vi "IPC Flasher Main.vi"() -> ()   [LabVIEW 2021]
uses:
  Controls/Console Manager Functions.ctl
  SubVIs/Global Variable.vi
panel:
  out "Console":string
  in  "Barcode":string="Barcode"
  in  "Run":bool
  in  "Stop":bool
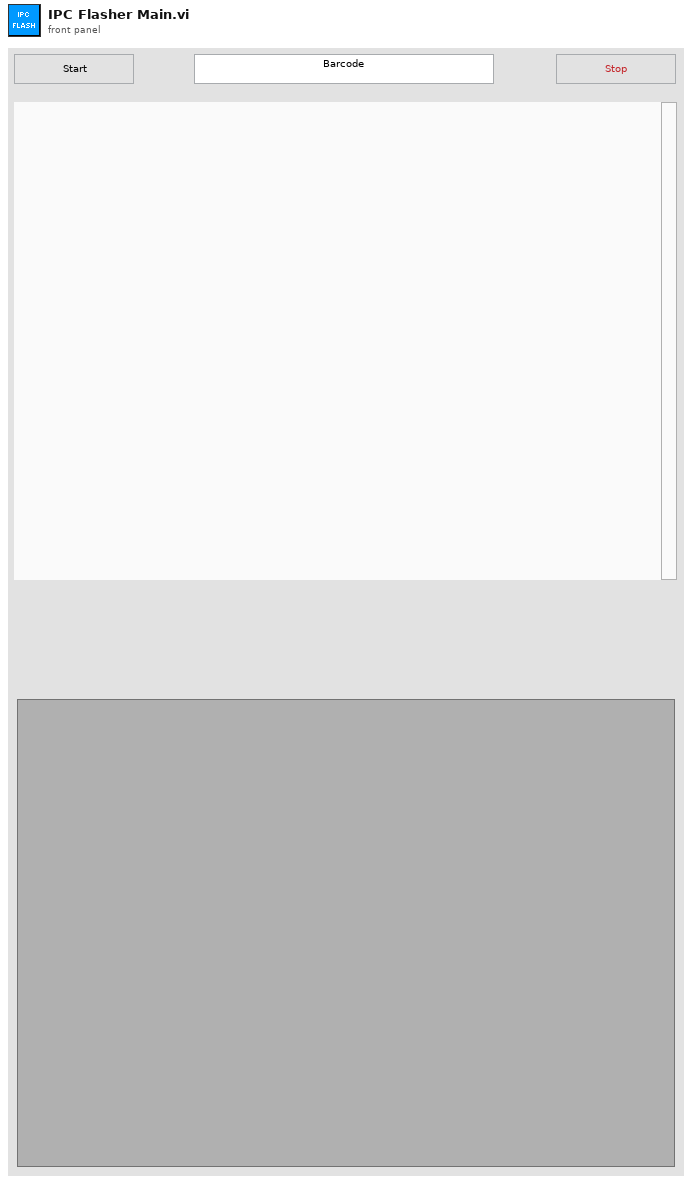
[diagram p1: front panel]
types:
  T1 = enum8{"Enabled", "Disabled", "Disabled and Grayed Out"}
  T2 = typedef "Console Manager Functions.ctl" = enum16{"Init", "Add", "Get"}
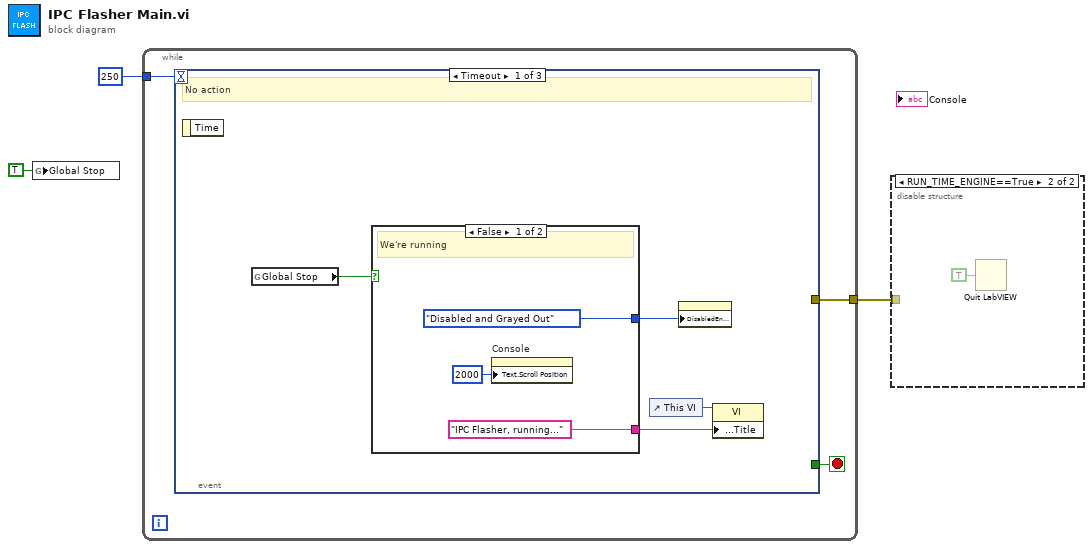
[diagram p0: block diagram]
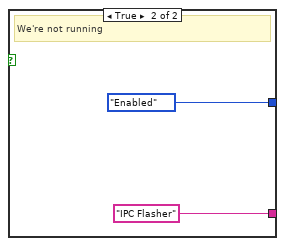
[diagram p3: hidden frame]
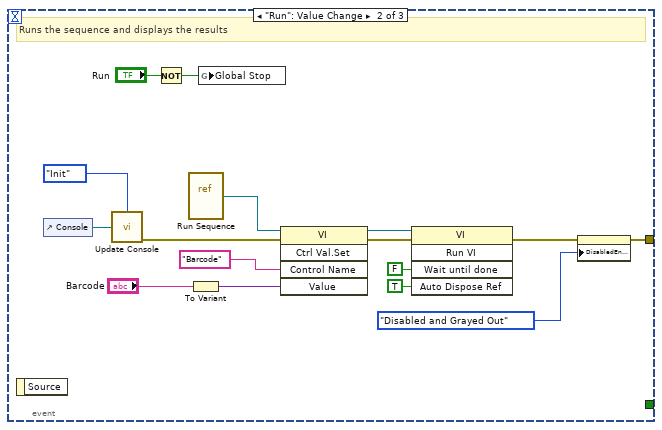
[diagram p4: hidden frame]
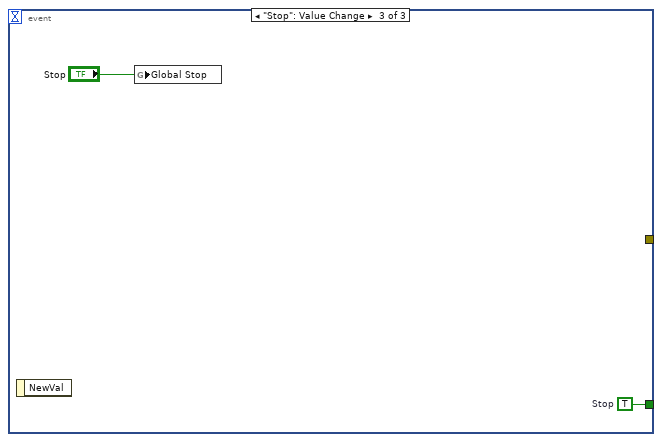
[diagram p5: hidden frame]
diagram:
  n1 = global write "Global Variable.vi" "Global Stop"(TRUE ("Global Stop")) -> ()
  n2 = while {
    tunnel: 250 -> [w6]
    tunnel: [w4] -> w2
    stop <- w5 stop-if-true
    n3 = event shown="[0] Timeout" {
      selector: _ -> [_ _ _]
      dyn-events: _ -> [_ _ _]
      timeout: w6 -> [_ _ _]
      tunnel: [_ _ w33] -> w5
      tunnel: [_ w21 _] -> w4
      event Timeout {
        # "No action"
        n4 = event-data() -> ()  [unwired: 1 in, 1 out]
        n5 = global read "Global Variable.vi" "Global Stop"() -> (w10:bool)
        n6 = case shown="False" w10 {
          tunnel: [T1."Disabled and Grayed Out" ("Disabled") T1."Enabled" ("Disabled")] -> w9
          tunnel: ["IPC Flasher, running..." ("Front Panel Window:Title") "IPC Flasher" ("Front Panel Window:Title")] -> w8
          frame False {
            # "We're running"
            n7 = property on="Console" class="Str"("Text.Scroll Position"=u32 2000) -> ()  [unwired: 2 in, 2 out]
          }
          frame True {
            # "We're not running"
          }
        }
        n8 = control-ref of="This VI"() -> (w7:refnum<vi>)
        n9 = property on="Run" class="Bool"("DisabledEnum"=w9) -> ()  [unwired: 2 in, 2 out]
        n10 = property class="VI"(reference=w7, "Front Panel.Title"=w8) -> ()  [unwired: 1 in, 2 out]
      }
      event "Run": Value Change {
        # "Runs the sequence and displays the results"
        n11 = event-data() -> ()  [unwired: 1 in, 1 out]
        n12 = control-ref of="Console"() -> (w18:refnum<vi>)
        n13 = call "Update Console.vi"("Function"=Console_Manager_Functions."Init", "Console Ref"=w18) -> ("Error Out"=w16:errorcluster)  [unwired: 12 in, 1 out]
        n14 = Not(x="Run") -> (.not. x?=w19:bool)
        n15 = vi-ref "Run Sequence.vi"() -> (w30:refnum<vi>)
        n16 = To Variant(anything="Barcode") -> (Variant=w27:variant)
        n17 = global write "Global Variable.vi" "Global Stop"(w19) -> ()
        n18 = invoke class="VI" method="Ctrl Val.Set"(reference=w30, error in=w16, "Control Name"="Barcode", "Value"=w27) -> (reference out=w26:refnum<vi>, error out=w25:errorcluster)  [unwired: 1 in, 3 out]
        n19 = invoke class="VI" method="Run VI"(reference=w26, error in=w25, "Wait until done"=FALSE ("Wait Until Done"), "Auto Dispose Ref"=TRUE ("Auto Dispose Reference")) -> (error out=w22:errorcluster)  [unwired: 1 in, 4 out]
        n20 = property on="Run" class="Bool"(error in=w22, "DisabledEnum"=T1."Disabled and Grayed Out" ("Disabled")) -> (error out=w21:errorcluster)  [unwired: 1 in, 1 out]
      }
      event "Stop": Value Change {
        w33 = TRUE  # Stop
        n21 = event-data() -> ()  [unwired: 1 in, 1 out]
        n22 = global write "Global Variable.vi" "Global Stop"("Stop") -> ()
      }
    }
  }
  n23 = disable-structure shown="RUN_TIME_ENGINE==True" {
    disable-tunnel: w2 -> [_ _]
    frame condition #0 (active) {
    }
    frame condition #1 {
      n24 = Quit LabVIEW(quit? (T)=TRUE) -> ()
    }
  }
